vi "Close test manager.vi"(5 "queueIDList":string[](array[string]), 6 "error in (no error)":errorcluster, 9 "Logger in":refnum<class "Logger.lvclass">) -> (0 "error out":errorcluster)   [LabVIEW 2026, in "Tests.lvlib"]
doc: "Shuts down the test LogManager via Logger.Shutdown, which stops every appender (each flushes and closes), and surfaces whether shutdown completed cleanly. Call after the test has dequeued and asserted on the capture queue. Fixture, not a test."
uses:
  Tests.lvlib
  src/Public/Logger.lvclass/Logger.lvclass
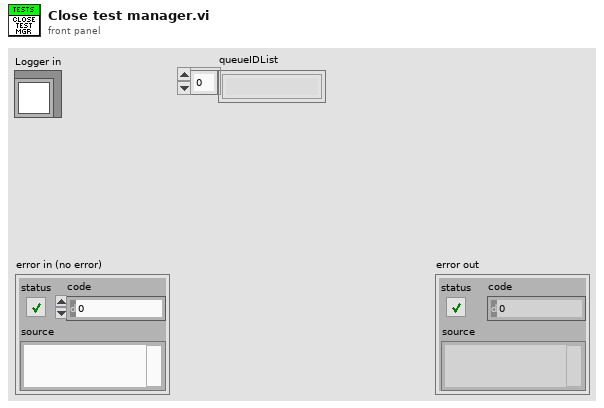
[diagram p1: front panel]
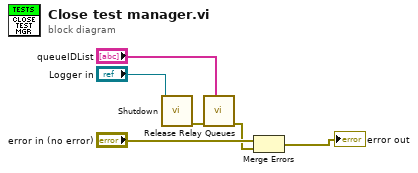
[diagram p0: block diagram]
diagram:
  n1 = call "Shutdown.vi"("Logger in"="Logger in") -> ("error out"=w5:errorcluster)  [unwired: 10 in]
  n2 = call "Release Relay Queues.vi"("queueIDList"="queueIDList", "error in (no error)"=w5) -> ("error out"=w2:errorcluster)  [unwired: 7 in]
  n3 = Merge Errors("error in (no error)", w2) -> (→"error out":errorcluster)
